vi "dynamics.vi"(0 "m":dbl, 1 "J_inv":T2 caption="Real Matrix", 2 "J":dbl[][](array[numeric]), 5 "r":dbl[](array[numeric]), 7 "E":cdb[](array[numeric]), 9 "W":dbl[](array[numeric]), 11 "M":cdb[](array[numeric]), 13 "q":dbl[](array[numeric])) -> (6 "W":dbl[](array[numeric]), 10 "unit quaternion":T1, 15 "E":dbl[](array[numeric]))   [LabVIEW 2018]
uses:
  <vilib>/Analysis/Matrix/Datatypes/RealMatrix.ctl
  <vilib>/robotics/Kinematics/Quaternion.ctl
  <vilib>/Analysis/coordinate.llb/Euler Rotation Order.ctl
  <vilib>/Analysis/_algsub.llb/Vector Norm.vi
  <vilib>/Analysis/_algsub.llb/Real Vector Norm.vi
  <vilib>/Analysis/baseanly.llb/Outer Product.vi
  <vilib>/Analysis/baseanly.llb/Real Outer Product.vi
  <vilib>/robotics/Kinematics/Create Lie Group Matrix.vi
  <vilib>/Analysis/Matrix/Numeric/Conversions/Matrix To Array - RM.vi
  <vilib>/imath/engines/lvmath2/RunTimeEngine/IndexRead/NIMS V(S).vi
  <instcachedir>/0/NIMS V(S)_0488751826AF41519A22953C041130DC.lvgen/NIMS V(S)_0488751826AF41519A22953C041130DC_003.vi
  <vilib>/imathl/engines/lvmath/Functions/Error Handling/Create Error.vi
  <vilib>/imath/engines/lvmath2/RunTimeEngine/BuiltInFunctions/cos/NIMS_cos(C).vi
  <instcachedir>/0/NIMS_cos(C)_96B8A70E6B8E4D29AD8526A89C8CF3DF.lvgen/NIMS_cos(C)_96B8A70E6B8E4D29AD8526A89C8CF3DF_001.vi
  <vilib>/imath/engines/lvmath2/RunTimeEngine/BuiltInFunctions/sin/NIMS_sin(C).vi
  <instcachedir>/0/NIMS_sin(C)_7FE83C8DCD97403BBE687635FA1F837E.lvgen/NIMS_sin(C)_7FE83C8DCD97403BBE687635FA1F837E_001.vi
  <vilib>/imath/engines/lvmath2/RunTimeEngine/BuiltInFunctions/reshapemx/NIMS_[GV]_reshapemx.vi
  <instcachedir>/0/NIMS_[GV]_reshapemx_FC3E9BFA29934BE8A99DD7B75AE8F89C.lvgen/NIMS_[GV]_reshapemx_FC3E9BFA29934BE8A99DD7B75AE8F89C_000.vi
  <instcachedir>/0/NIMS V(S)_0488751826AF41519A22953C041130DC.lvgen/NIMS V(S)_0488751826AF41519A22953C041130DC_000.vi
  <vilib>/imath/engines/lvmath2/RunTimeEngine/ArithmeticOperatorToken/NIMS_ArithmeticOperator_multmx.vi
  <instcachedir>/0/NIMS_ArithmeticOperator_multmx_622CA76F9646436AB036D42A9A1CE0E6.lvgen/NIMS_ArithmeticOperator_multmx_622CA76F9646436AB036D42A9A1CE0E6_004.vi
  <vilib>/imath/engines/lvmath2/RunTimeEngine/ArithmeticOperatorToken/NIMS_ArithmeticOperator_multmx(M,CV).vi
  <instcachedir>/0/NIMS_ArithmeticOperator_multmx(M,CV)_2F1CD6A2FE4F4213A4AD1C901C2750F5.lvgen/NIMS_ArithmeticOperator_multmx(M,CV)_2F1CD6A2FE4F4213A4AD1C901C2750F5_000.vi
  <vilib>/imath/engines/lvmath2/RunTimeEngine/ErrorHandling/NIMS_Create Error From Enums.vi
  <vilib>/imath/engines/lvmath2/RunTimeEngine/ArithmeticOperatorToken/NIMS_ArithmeticOperator_multmx(M,CV)-internal.vi
  <instcachedir>/0/NIMS_ArithmeticOperator_multmx(M,CV)-internal_5287250D8D1D4A3E9F77F5DF08D432E0.lvgen/NIMS_ArithmeticOperator_multmx(M,CV)-internal_5287250D8D1D4A3E9F77F5DF08D432E0_004.vi
  <vilib>/imath/engines/lvmath2/RunTimeEngine/ArithmeticOperatorToken/NIMS_ArithmeticOperator_minus.vi
  <instcachedir>/0/NIMS_ArithmeticOperator_minus_C4D0373119CC411691B2E50DF2E09F22.lvgen/NIMS_ArithmeticOperator_minus_C4D0373119CC411691B2E50DF2E09F22_000.vi
  <instcachedir>/0/NIMS_ArithmeticOperator_minus_C4D0373119CC411691B2E50DF2E09F22.lvgen/NIMS_ArithmeticOperator_minus_C4D0373119CC411691B2E50DF2E09F22_009.vi
  <instcachedir>/0/NIMS_ArithmeticOperator_multmx_622CA76F9646436AB036D42A9A1CE0E6.lvgen/NIMS_ArithmeticOperator_multmx_622CA76F9646436AB036D42A9A1CE0E6_008.vi
  <vilib>/imath/engines/lvmath2/RunTimeEngine/IndexRead/NIMS M(S).vi
  <instcachedir>/0/NIMS M(S)_B826C018497E4940AE96BD27B540B6FB.lvgen/NIMS M(S)_B826C018497E4940AE96BD27B540B6FB_004.vi
  <vilib>/imath/engines/lvmath2/RunTimeEngine/NodeEndStatement/NIMS_NodeEndStatement_Output.vi
  <instcachedir>/0/NIMS_NodeEndStatement_Output_53EC0D466D134D7ABD903AC30B43404B.lvgen/NIMS_NodeEndStatement_Output_53EC0D466D134D7ABD903AC30B43404B_005.vi
  <vilib>/imath/engines/lvmath2/RunTimeEngine/ErrorHandling/NIMS_Finalize Error.vi
  <vilib>/imath/engines/lvmath2/RunTimeEngine/Managers/WorkSpace/UID Generator.vi
  <vilib>/imath/engines/lvmath2/RunTimeEngine/RunTimeType/NIMS_RunTimeType_From StrictType (excl LVString).vi
  <instcachedir>/0/NIMS_RunTimeType_From StrictType (excl LVString)_E7E34A65C99947108168652BAD14964D.lvgen/NIMS_RunTimeType_From StrictType (excl LVString)_E7E34A65C99947108168652BAD14964D_000.vi
  <vilib>/imath/engines/lvmath2/RunTimeEngine/LocalVariableDefStatement/MC_LocalVariableDefStatement_Display.vi
  <instcachedir>/0/NIMS M(S)_B826C018497E4940AE96BD27B540B6FB.lvgen/NIMS M(S)_B826C018497E4940AE96BD27B540B6FB_000.vi
  <vilib>/imath/engines/lvmath2/RunTimeEngine/Managers/SymbolTable/Clear UID.vi
  <vilib>/Analysis/Matrix/Numeric/Multiply/Multiply.vi
  <vilib>/Analysis/Matrix/Numeric/Multiply/Multiply - RM,R.vi
  <vilib>/Analysis/Matrix/Numeric/Multiply/Multiply - R,RM.vi
  <vilib>/Analysis/Matrix/Numeric/Add/Add.vi
  <vilib>/Analysis/Matrix/Numeric/Add/Add - RM,RM.vi
  <vilib>/gmath/NI_Gmath.lvlib
  <vilib>/imath/engines/lvmath2/RunTimeEngine/Managers/SymbolTable/NIMS_WorkSpace.lvlib
  <vilib>/robotics/Kinematics/NI_Kinematics.lvlib
  <vilib>/Analysis/NI_AALPro.lvlib
  <vilib>/Analysis/Matrix/NI_Matrix.lvlib
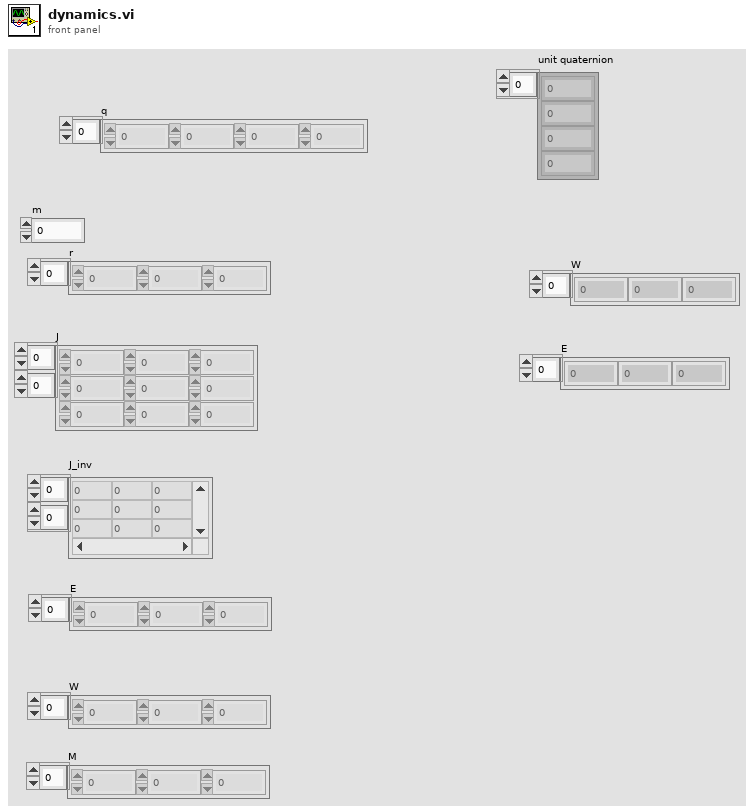
[diagram p1: front panel]
types:
  T1 = typedef "NI_Kinematics.lvlib/Quaternion.ctl" = dbl[]
  T2 = typedef "NI_Matrix.lvlib/RealMatrix.ctl" = dbl[][]
  T3 = typedef "NI_AALPro.lvlib/Euler Rotation Order.ctl" = u16
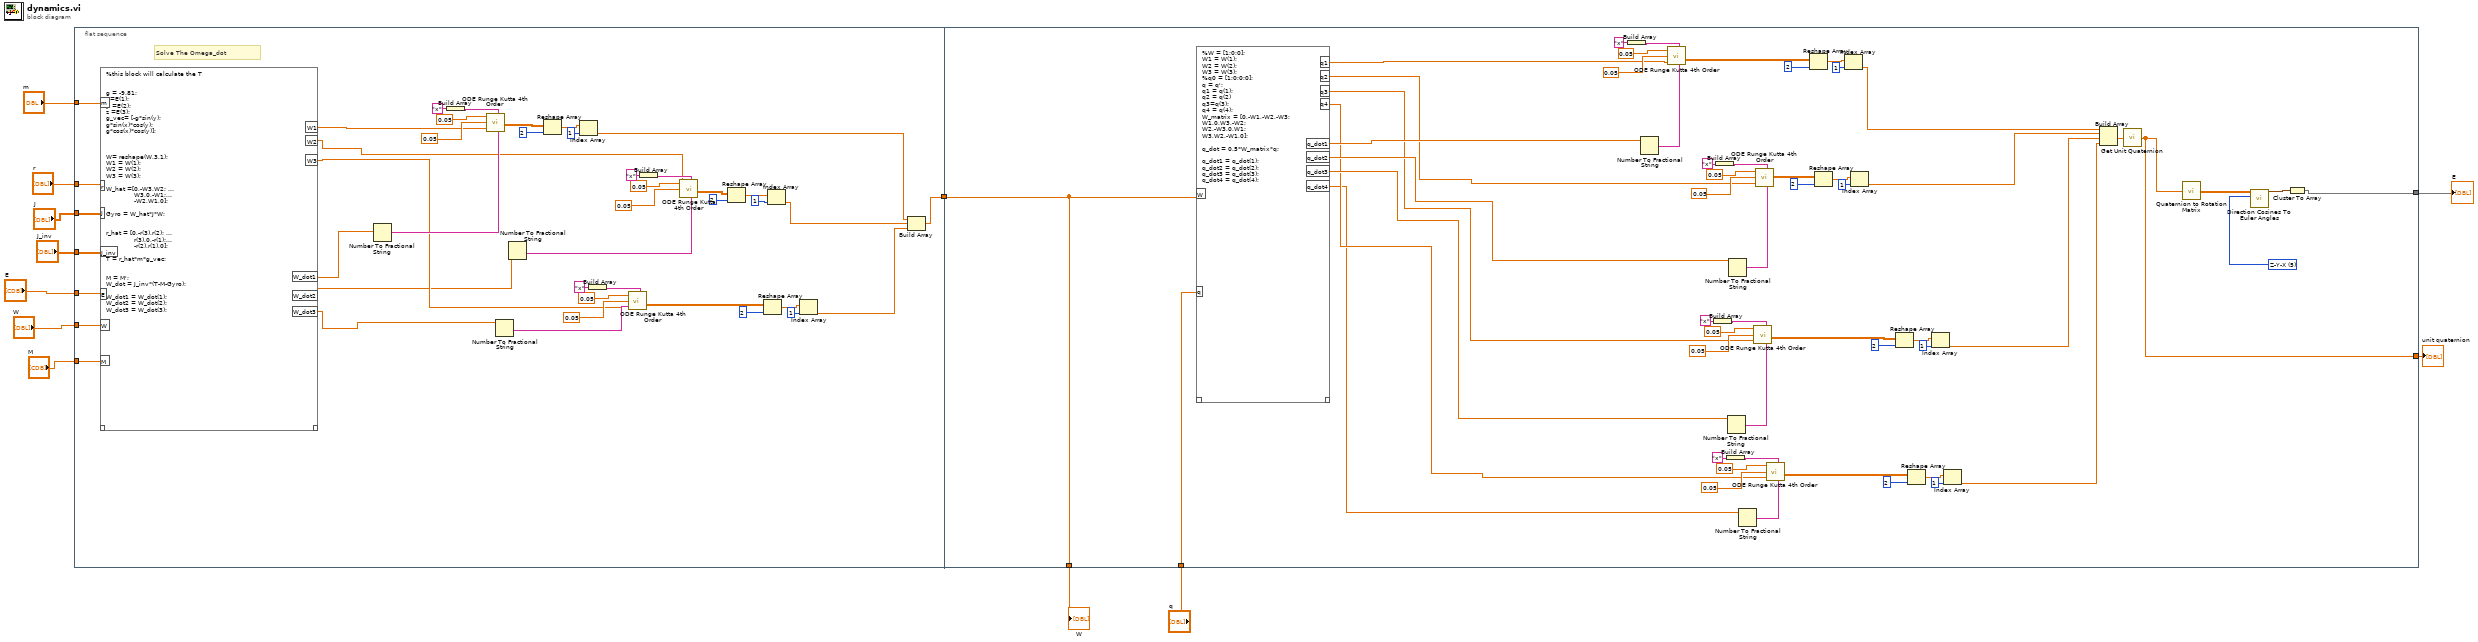
[diagram p0: block diagram]
diagram:
  n1 = flat-sequence {
    tunnel: [w20] -> w12
    tunnel: "m" -> [w19]
    tunnel: "r" -> [w18]
    tunnel: "J" -> [w17]
    tunnel: "J_inv" -> [w16]
    tunnel: "E" -> [w15]
    tunnel: "W" -> [w14]
    tunnel: "M" -> [w13]
    tunnel: w12 -> [w496]
    tunnel: [w496] -> w11
    tunnel: [w494] -> w10
    tunnel: "q" -> [w493]
    tunnel: [w492] -> w1
    frame #0 {
      # "Solve The Omega_dot"
      n2 = mathscript code="%this block will calculate the T\n\n\ng = -9.81;\nx=E(1);\ny =E(2);\nz =E(3);\ng_vec= [-g*sin(y);\ng*sin(x)*cos(y);\ng*cos(x)*cos(y)];\n\n\n\nW= reshape(W,3,1);\nW1 = W(1);\nW2 = W(2);\nW3 = W(3);\n\nW_hat =[0,-W3,W2; ...\n              W3,0,-W1;...\n              -W2,W1,0];\n\nGyro = W_hat*J*W;\n\n\nr_hat = [0,-r(3),r(2); ...\n              r(3),0,-r(1);...\n              -r(2),r(1),0];\n\nT = r_hat*m*g_vec;\n\n\nM = M';\nW_dot = J_inv*(T-M-Gyro);\n\nW_dot1 = W_dot(1);\nW_dot2 = W_dot(2);\nW_dot3 = W_dot(3);"("E"=w15, "J"=w17, "J_inv"=w16, "r"=w18, "m"=w19, "W"=w14, "M"=w13) -> ("W_dot1"=w21:dbl[], "W_dot2"=w22:dbl[], "W_dot3"=w23:dbl[], "W1"=w26:dbl[], "W2"=w25:dbl[], "W3"=w24:dbl[])  [unwired: 1 in, 1 out]
      n3 = Number To Fractional String(number=w21) -> (F-format string=w52:string[])  [unwired: 3 in]
      n4 = Build Array("x") -> (w55:string[])
      n5 = call <vilib>:"ODE Runge Kutta 4th Order.vi"("time end"=0.05, "h (step rate)"=0.05, "X0"=w26, "X (name of variables)"=w55, "F(X,t) (right sides of the ODE\nas functions of X and t)"=w52) -> ("X Values (solution)"=w48:dbl[][])  [unwired: 2 in, 3 out]
      n6 = Number To Fractional String(number=w23) -> (F-format string=w34:string[])  [unwired: 3 in]
      n7 = Number To Fractional String(number=w22) -> (F-format string=w43:string[])  [unwired: 3 in]
      n8 = Reshape Array(w48, 2 ("dimension size")) -> (w50:dbl[])
      n9 = Index Array(array=w50, index=1) -> (element=w29:dbl)
      n10 = Build Array("x") -> (w37:string[])
      n11 = call <vilib>:"ODE Runge Kutta 4th Order.vi"("time end"=0.05, "h (step rate)"=0.05, "X0"=w24, "X (name of variables)"=w37, "F(X,t) (right sides of the ODE\nas functions of X and t)"=w34) -> ("X Values (solution)"=w30:dbl[][])  [unwired: 2 in, 3 out]
      n12 = Build Array("x") -> (w46:string[])
      n13 = call <vilib>:"ODE Runge Kutta 4th Order.vi"("time end"=0.05, "h (step rate)"=0.05, "X0"=w25, "X (name of variables)"=w46, "F(X,t) (right sides of the ODE\nas functions of X and t)"=w43) -> ("X Values (solution)"=w39:dbl[][])  [unwired: 2 in, 3 out]
      n14 = Reshape Array(w39, 2 ("dimension size")) -> (w41:dbl[])
      n15 = Reshape Array(w30, 2 ("dimension size")) -> (w32:dbl[])
      n16 = Index Array(array=w41, index=1) -> (element=w28:dbl)
      n17 = Index Array(array=w32, index=1) -> (element=w27:dbl)
      n18 = Build Array(w29, w28, w27) -> (w20:dbl[])
    }
    frame #1 {
      w497 = T3 5 items=["X-Y-Z", "X-Z-Y", "Y-X-Z", "Y-Z-X", "Z-X-Y", "Z-Y-X", "X-Y-X", "X-Z-X", "Y-X-Y", "Y-Z-Y", "Z-X-Z", "Z-Y-Z"] ("rotation order")
      n19 = mathscript code="%W = [1;0;0];\nW1 = W(1);\nW2 = W(2);\nW3 = W(3);\n%q0 = [1;0;0;0];\nq = q';\nq1 = q(1);\nq2 = q(2)\nq3=q(3);\nq4 = q(4);\nW_matrix = [0,-W1,-W2,-W3;\nW1,0,W3,-W2;\nW2,-W3,0,W1;\nW3,W2,-W1,0];\n\nq_dot = 0.5*W_matrix*q;\n\nq_dot1 = q_dot(1);\nq_dot2 = q_dot(2);\nq_dot3 = q_dot(3);\nq_dot4 = q_dot(4);"("q"=w493, "W"=w496) -> ("q_dot1"=w537:dbl[], "q_dot2"=w526:dbl[], "q_dot3"=w515:dbl[], "q_dot4"=w504:dbl[], "q1"=w538:dbl[], "q2"=w527:dbl[], "q3"=w516:dbl[], "q4"=w505:dbl[])  [unwired: 1 in, 1 out]
      n20 = Build Array("x") -> (w546:string[])
      n21 = Number To Fractional String(number=w537) -> (F-format string=w543:string[])  [unwired: 3 in]
      n22 = call <vilib>:"ODE Runge Kutta 4th Order.vi"("time end"=0.05, "h (step rate)"=0.05, "X0"=w538, "X (name of variables)"=w546, "F(X,t) (right sides of the ODE\nas functions of X and t)"=w543) -> ("X Values (solution)"=w539:dbl[][])  [unwired: 2 in, 3 out]
      n23 = Build Array("x") -> (w524:string[])
      n24 = Build Array("x") -> (w535:string[])
      n25 = Build Array("x") -> (w513:string[])
      n26 = Number To Fractional String(number=w515) -> (F-format string=w521:string[])  [unwired: 3 in]
      n27 = Number To Fractional String(number=w526) -> (F-format string=w532:string[])  [unwired: 3 in]
      n28 = Number To Fractional String(number=w504) -> (F-format string=w510:string[])  [unwired: 3 in]
      n29 = call <vilib>:"ODE Runge Kutta 4th Order.vi"("time end"=0.05, "h (step rate)"=0.05, "X0"=w516, "X (name of variables)"=w524, "F(X,t) (right sides of the ODE\nas functions of X and t)"=w521) -> ("X Values (solution)"=w517:dbl[][])  [unwired: 2 in, 3 out]
      n30 = call <vilib>:"ODE Runge Kutta 4th Order.vi"("time end"=0.05, "h (step rate)"=0.05, "X0"=w527, "X (name of variables)"=w535, "F(X,t) (right sides of the ODE\nas functions of X and t)"=w532) -> ("X Values (solution)"=w528:dbl[][])  [unwired: 2 in, 3 out]
      n31 = call <vilib>:"ODE Runge Kutta 4th Order.vi"("time end"=0.05, "h (step rate)"=0.05, "X0"=w505, "X (name of variables)"=w513, "F(X,t) (right sides of the ODE\nas functions of X and t)"=w510) -> ("X Values (solution)"=w506:dbl[][])  [unwired: 2 in, 3 out]
      n32 = Reshape Array(w539, 2 ("dimension size")) -> (w541:dbl[])
      n33 = Reshape Array(w528, 2 ("dimension size")) -> (w530:dbl[])
      n34 = Index Array(array=w541, index=1) -> (element=w503:dbl)
      n35 = Index Array(array=w530, index=1) -> (element=w502:dbl)
      n36 = Reshape Array(w517, 2 ("dimension size")) -> (w519:dbl[])
      n37 = Reshape Array(w506, 2 ("dimension size")) -> (w508:dbl[])
      n38 = Index Array(array=w519, index=1) -> (element=w501:dbl)
      n39 = Index Array(array=w508, index=1) -> (element=w500:dbl)
      n40 = Build Array(w503, w502, w501, w500) -> (w499:dbl[])
      n41 = call <vilib>:"Get Unit Quaternion.vi"("quaternion"=w499) -> ("unit quaternion"=w492:T1)
      n42 = call <vilib>:"Quaternion to Rotation Matrix.vi"("quaternion"=w492) -> ("rotation matrix"=w498:T2)
      n43 = call <vilib>:"Direction Cosines To Euler Angles.vi"("rotation order"=w497, "Direction Cosines"=w498) -> ("Euler Angles"=w495:cluster{"phi":dbl, "theta":dbl, "psi":dbl})  [unwired: 8 in, 1 out]
      n44 = Cluster To Array(cluster=w495) -> (array=w494:dbl[])
    }
  }
  "W" <- w11
  "E" <- w10
  "unit quaternion" <- w1
